vi "calculator.vi"() -> ()   [LabVIEW 2019]
panel:
  in  "Decimal Point Places":i16
  out "Previous Display":string
  in  ".":bool
  in  "=":bool
  in  "Clear":bool
  in  "Exit":bool
  out "Current Display":string
  in  "+":bool
  in  "-":bool
  in  "/":bool
  in  "x":bool
  in  "9":bool
  in  "8":bool
  in  "7":bool
  in  "6":bool
  in  "5":bool
  in  "4":bool
  in  "3":bool
  in  "0":bool
  in  "2":bool
  in  "1":bool
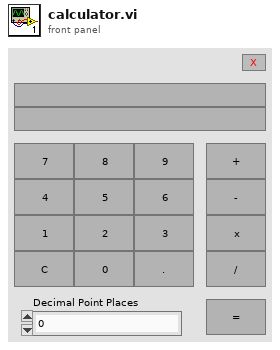
[diagram p1: front panel]
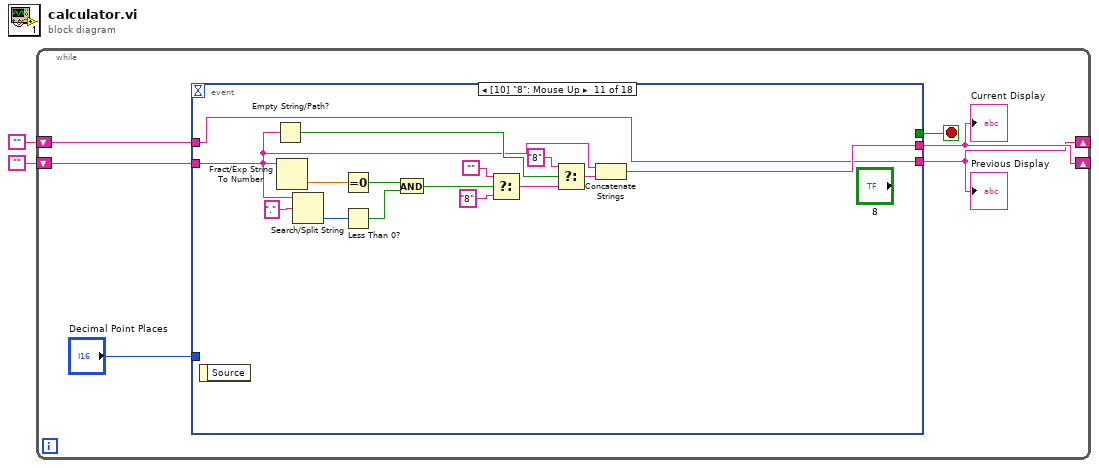
[diagram p0: block diagram]
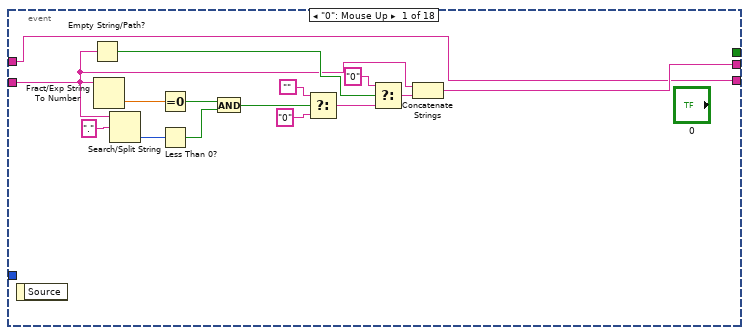
[diagram p2: hidden frame]
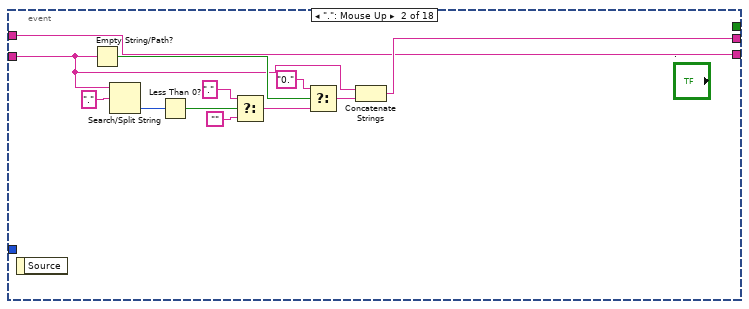
[diagram p3: hidden frame]
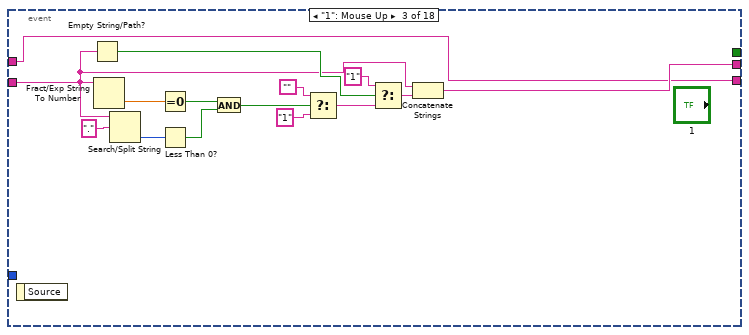
[diagram p4: hidden frame]
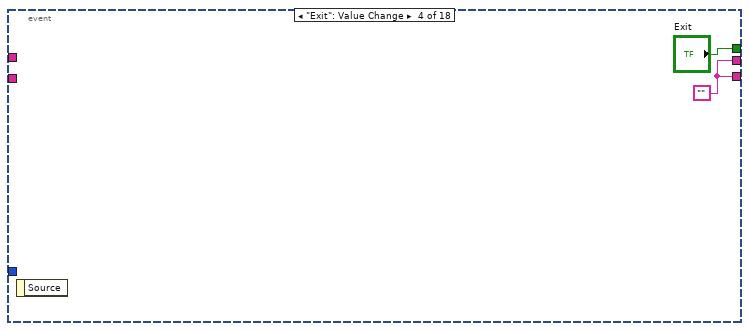
[diagram p5: hidden frame]
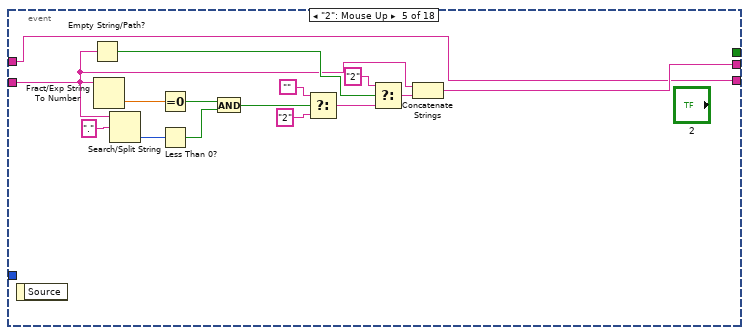
[diagram p6: hidden frame]
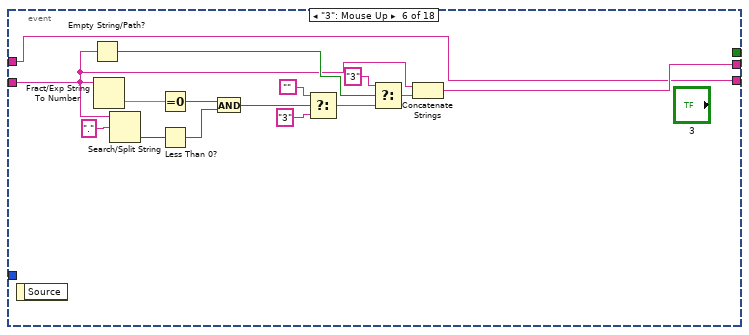
[diagram p7: hidden frame]
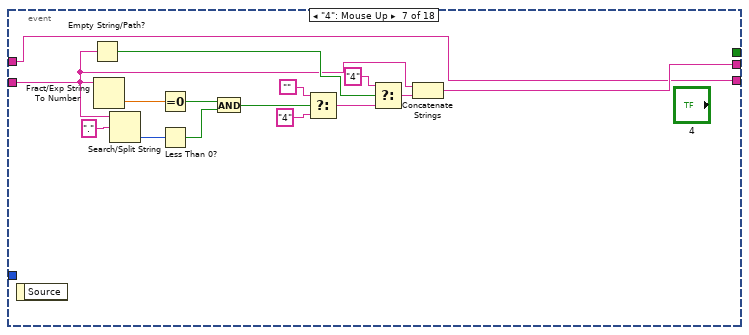
[diagram p8: hidden frame]
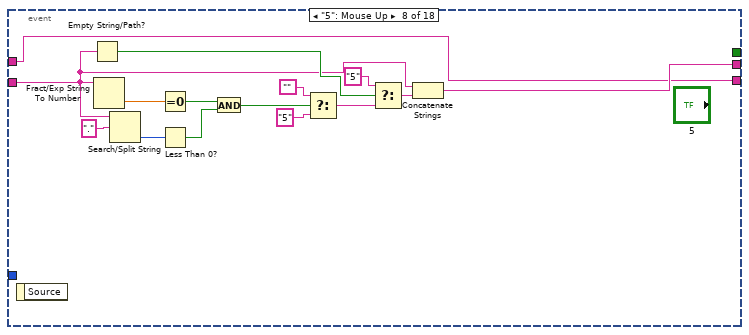
[diagram p9: hidden frame]
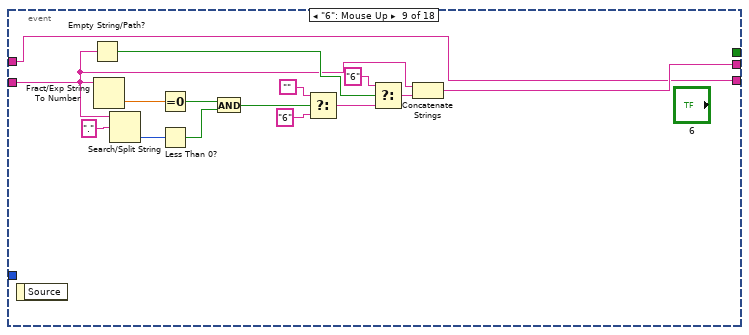
[diagram p10: hidden frame]
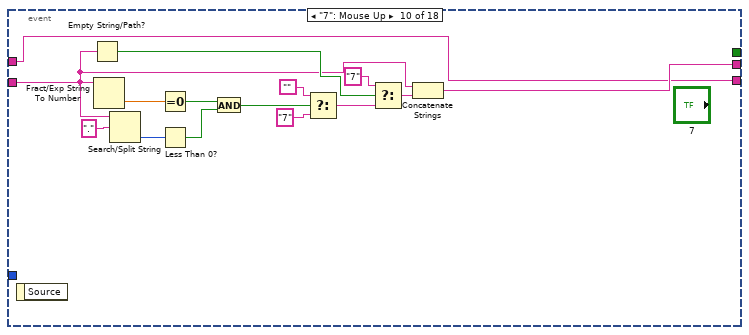
[diagram p11: hidden frame]
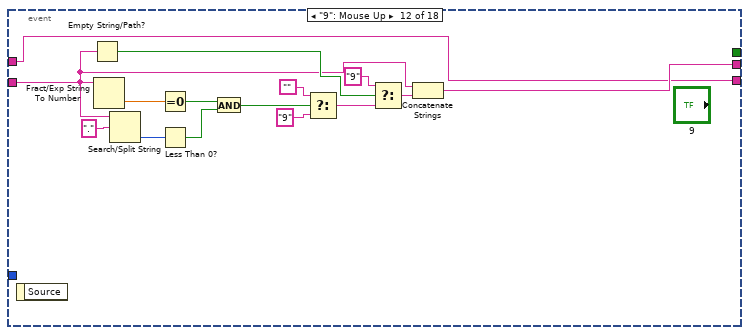
[diagram p12: hidden frame]
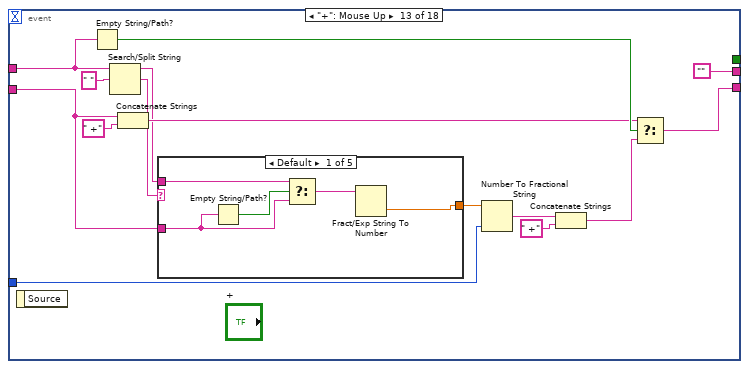
[diagram p13: hidden frame]
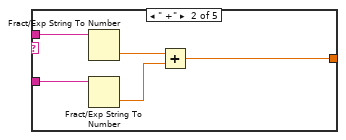
[diagram p14: hidden frame]
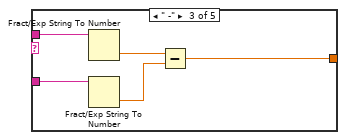
[diagram p15: hidden frame]
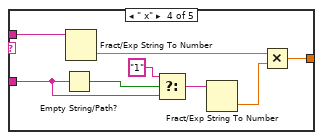
[diagram p16: hidden frame]
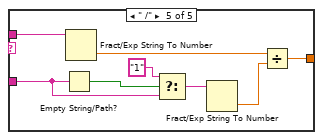
[diagram p17: hidden frame]
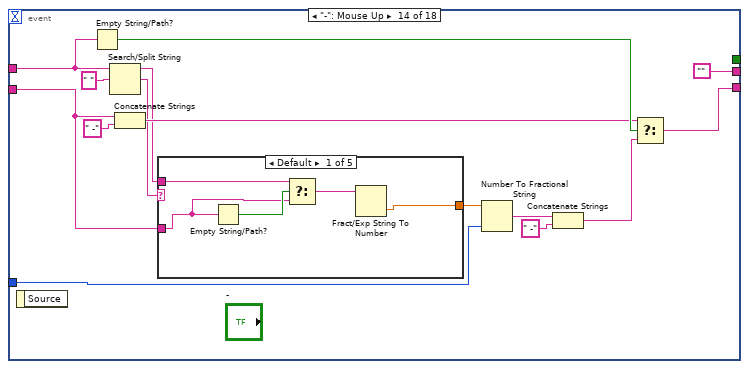
[diagram p18: hidden frame]
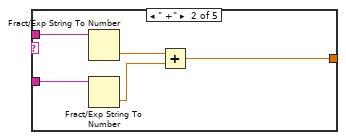
[diagram p19: hidden frame]
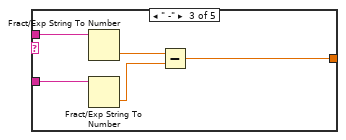
[diagram p20: hidden frame]
diagram:
  n1 = while {
    shift-right: [w8] -> _
    shift-left: "" -> [w7]
    shift-right: [w5] -> _
    shift-left: "" -> [w4]
    stop <- w6 stop-if-true
    n2 = event shown="[10] \"8\": Mouse Up" {
      selector: _ -> [_ _ _ _ _ _ _ _ _ _ _ _ _ _ _ _ _ _]
      dyn-events: _ -> [_ _ _ _ _ _ _ _ _ _ _ _ _ _ _ _ _ _]
      timeout: _ -> [_ _ _ _ _ _ _ _ _ _ _ _ _ _ _ _ _ _]
      tunnel: [w17 w27 w44 w51 w60 w75 w90 w105 w120 w135 w150 w165 "" "" "" "" "" w401] -> w8
      tunnel: w7 -> [w14 w28 w38 _ w55 w70 w85 w100 w115 w130 w145 w160 w174 w223 w271 w313 w358 _]
      tunnel: [_ _ _ "Exit" _ _ _ _ _ _ _ _ _ _ _ _ _ _] -> w6
      tunnel: [w15 w24 w42 w51 w59 w74 w89 w104 w119 w134 w149 w164 w184 w228 w270 w320 w360 w401] -> w5
      tunnel: w4 -> [w15 w24 w42 _ w59 w74 w89 w104 w119 w134 w149 w164 w183 w229 w272 w321 w359 _]
      tunnel: "Decimal Point Places" -> [_ _ _ _ _ _ _ _ _ _ _ _ w173 w219 w265 w311 w357 _]
      event "0": Mouse Up {
        n3 = event-data() -> ()  [unwired: 1 in, 1 out]
        n4 = Empty String/Path?(string/path=w14) -> (empty?=w23:bool)
        n5 = Fract/Exp String To Number(string=w14) -> (number=w21:dbl)  [unwired: 3 in, 1 out]
        n6 = Search/Split String(string=w14, search string/char (-)=".") -> (offset of match=w12:i32)  [unwired: 1 in, 2 out]
        n7 = Equal To 0?(x=w21) -> (x = 0?=w11:bool)
        n8 = Less Than 0?(x=w12) -> (x < 0?=w10:bool)
        n9 = And(x=w11, y=w10) -> (x .and. y?=w9:bool)
        n10 = Select(t="", s=w9, f="0") -> (s? t:f=w18:string)
        n11 = Select(t="0", s=w23, f=w18) -> (s? t:f=w16:string)
        n12 = Concatenate Strings(w14, w16) -> (w17:string)
      }
      event ".": Mouse Up {
        n13 = event-data() -> ()  [unwired: 1 in, 1 out]
        n14 = Empty String/Path?(string/path=w28) -> (empty?=w35:bool)
        n15 = Search/Split String(string=w28, search string/char (-)=".") -> (offset of match=w32:i32)  [unwired: 1 in, 2 out]
        n16 = Less Than 0?(x=w32) -> (x < 0?=w31:bool)
        n17 = Select(t=".", s=w31, f="") -> (s? t:f=w30:string)
        n18 = Select(t="0.", s=w35, f=w30) -> (s? t:f=w29:string)
        n19 = Concatenate Strings(w28, w29) -> (w27:string)
      }
      event "1": Mouse Up {
        n20 = event-data() -> ()  [unwired: 1 in, 1 out]
        n21 = Empty String/Path?(string/path=w38) -> (empty?=w50:bool)
        n22 = Fract/Exp String To Number(string=w38) -> (number=w49:dbl)  [unwired: 3 in, 1 out]
        n23 = Search/Split String(string=w38, search string/char (-)=".") -> (offset of match=w40:i32)  [unwired: 1 in, 2 out]
        n24 = Equal To 0?(x=w49) -> (x = 0?=w37:bool)
        n25 = Less Than 0?(x=w40) -> (x < 0?=w39:bool)
        n26 = And(x=w37, y=w39) -> (x .and. y?=w36:bool)
        n27 = Select(t="", s=w36, f="1") -> (s? t:f=w46:string)
        n28 = Select(t="1", s=w50, f=w46) -> (s? t:f=w43:string)
        n29 = Concatenate Strings(w38, w43) -> (w44:string)
      }
      event "Exit": Value Change {
        w51 = ""
        n30 = event-data() -> ()  [unwired: 1 in, 1 out]
      }
      event "2": Mouse Up {
        n31 = event-data() -> ()  [unwired: 1 in, 1 out]
        n32 = Empty String/Path?(string/path=w55) -> (empty?=w67:bool)
        n33 = Fract/Exp String To Number(string=w55) -> (number=w65:dbl)  [unwired: 3 in, 1 out]
        n34 = Search/Split String(string=w55, search string/char (-)=".") -> (offset of match=w57:i32)  [unwired: 1 in, 2 out]
        n35 = Equal To 0?(x=w65) -> (x = 0?=w54:bool)
        n36 = Less Than 0?(x=w57) -> (x < 0?=w56:bool)
        n37 = And(x=w54, y=w56) -> (x .and. y?=w53:bool)
        n38 = Select(t="", s=w53, f="2") -> (s? t:f=w62:string)
        n39 = Select(t="2", s=w67, f=w62) -> (s? t:f=w61:string)
        n40 = Concatenate Strings(w55, w61) -> (w60:string)
      }
      event "3": Mouse Up {
        n41 = event-data() -> ()  [unwired: 1 in, 1 out]
        n42 = Empty String/Path?(string/path=w70) -> (empty?=w82:bool)
        n43 = Fract/Exp String To Number(string=w70) -> (number=w80:dbl)  [unwired: 3 in, 1 out]
        n44 = Search/Split String(string=w70, search string/char (-)=".") -> (offset of match=w72:i32)  [unwired: 1 in, 2 out]
        n45 = Equal To 0?(x=w80) -> (x = 0?=w69:bool)
        n46 = Less Than 0?(x=w72) -> (x < 0?=w71:bool)
        n47 = And(x=w69, y=w71) -> (x .and. y?=w68:bool)
        n48 = Select(t="", s=w68, f="3") -> (s? t:f=w77:string)
        n49 = Select(t="3", s=w82, f=w77) -> (s? t:f=w76:string)
        n50 = Concatenate Strings(w70, w76) -> (w75:string)
      }
      event "4": Mouse Up {
        n51 = event-data() -> ()  [unwired: 1 in, 1 out]
        n52 = Empty String/Path?(string/path=w85) -> (empty?=w97:bool)
        n53 = Fract/Exp String To Number(string=w85) -> (number=w95:dbl)  [unwired: 3 in, 1 out]
        n54 = Search/Split String(string=w85, search string/char (-)=".") -> (offset of match=w87:i32)  [unwired: 1 in, 2 out]
        n55 = Equal To 0?(x=w95) -> (x = 0?=w84:bool)
        n56 = Less Than 0?(x=w87) -> (x < 0?=w86:bool)
        n57 = And(x=w84, y=w86) -> (x .and. y?=w83:bool)
        n58 = Select(t="", s=w83, f="4") -> (s? t:f=w92:string)
        n59 = Select(t="4", s=w97, f=w92) -> (s? t:f=w91:string)
        n60 = Concatenate Strings(w85, w91) -> (w90:string)
      }
      event "5": Mouse Up {
        n61 = event-data() -> ()  [unwired: 1 in, 1 out]
        n62 = Empty String/Path?(string/path=w100) -> (empty?=w112:bool)
        n63 = Fract/Exp String To Number(string=w100) -> (number=w110:dbl)  [unwired: 3 in, 1 out]
        n64 = Search/Split String(string=w100, search string/char (-)=".") -> (offset of match=w102:i32)  [unwired: 1 in, 2 out]
        n65 = Equal To 0?(x=w110) -> (x = 0?=w99:bool)
        n66 = Less Than 0?(x=w102) -> (x < 0?=w101:bool)
        n67 = And(x=w99, y=w101) -> (x .and. y?=w98:bool)
        n68 = Select(t="", s=w98, f="5") -> (s? t:f=w107:string)
        n69 = Select(t="5", s=w112, f=w107) -> (s? t:f=w106:string)
        n70 = Concatenate Strings(w100, w106) -> (w105:string)
      }
      event "6": Mouse Up {
        n71 = event-data() -> ()  [unwired: 1 in, 1 out]
        n72 = Empty String/Path?(string/path=w115) -> (empty?=w127:bool)
        n73 = Fract/Exp String To Number(string=w115) -> (number=w125:dbl)  [unwired: 3 in, 1 out]
        n74 = Search/Split String(string=w115, search string/char (-)=".") -> (offset of match=w117:i32)  [unwired: 1 in, 2 out]
        n75 = Equal To 0?(x=w125) -> (x = 0?=w114:bool)
        n76 = Less Than 0?(x=w117) -> (x < 0?=w116:bool)
        n77 = And(x=w114, y=w116) -> (x .and. y?=w113:bool)
        n78 = Select(t="", s=w113, f="6") -> (s? t:f=w122:string)
        n79 = Select(t="6", s=w127, f=w122) -> (s? t:f=w121:string)
        n80 = Concatenate Strings(w115, w121) -> (w120:string)
      }
      event "7": Mouse Up {
        n81 = event-data() -> ()  [unwired: 1 in, 1 out]
        n82 = Empty String/Path?(string/path=w130) -> (empty?=w142:bool)
        n83 = Fract/Exp String To Number(string=w130) -> (number=w140:dbl)  [unwired: 3 in, 1 out]
        n84 = Search/Split String(string=w130, search string/char (-)=".") -> (offset of match=w132:i32)  [unwired: 1 in, 2 out]
        n85 = Equal To 0?(x=w140) -> (x = 0?=w129:bool)
        n86 = Less Than 0?(x=w132) -> (x < 0?=w131:bool)
        n87 = And(x=w129, y=w131) -> (x .and. y?=w128:bool)
        n88 = Select(t="", s=w128, f="7") -> (s? t:f=w137:string)
        n89 = Select(t="7", s=w142, f=w137) -> (s? t:f=w136:string)
        n90 = Concatenate Strings(w130, w136) -> (w135:string)
      }
      event "8": Mouse Up {
        n91 = event-data() -> ()  [unwired: 1 in, 1 out]
        n92 = Empty String/Path?(string/path=w145) -> (empty?=w157:bool)
        n93 = Fract/Exp String To Number(string=w145) -> (number=w155:dbl)  [unwired: 3 in, 1 out]
        n94 = Search/Split String(string=w145, search string/char (-)=".") -> (offset of match=w147:i32)  [unwired: 1 in, 2 out]
        n95 = Equal To 0?(x=w155) -> (x = 0?=w144:bool)
        n96 = Less Than 0?(x=w147) -> (x < 0?=w146:bool)
        n97 = And(x=w144, y=w146) -> (x .and. y?=w143:bool)
        n98 = Select(t="", s=w143, f="8") -> (s? t:f=w152:string)
        n99 = Select(t="8", s=w157, f=w152) -> (s? t:f=w151:string)
        n100 = Concatenate Strings(w145, w151) -> (w150:string)
      }
      event "9": Mouse Up {
        n101 = event-data() -> ()  [unwired: 1 in, 1 out]
        n102 = Empty String/Path?(string/path=w160) -> (empty?=w172:bool)
        n103 = Fract/Exp String To Number(string=w160) -> (number=w170:dbl)  [unwired: 3 in, 1 out]
        n104 = Search/Split String(string=w160, search string/char (-)=".") -> (offset of match=w162:i32)  [unwired: 1 in, 2 out]
        n105 = Equal To 0?(x=w170) -> (x = 0?=w159:bool)
        n106 = Less Than 0?(x=w162) -> (x < 0?=w161:bool)
        n107 = And(x=w159, y=w161) -> (x .and. y?=w158:bool)
        n108 = Select(t="", s=w158, f="9") -> (s? t:f=w167:string)
        n109 = Select(t="9", s=w172, f=w167) -> (s? t:f=w166:string)
        n110 = Concatenate Strings(w160, w166) -> (w165:string)
      }
      event "+": Mouse Up {
        n111 = event-data() -> ()  [unwired: 1 in, 1 out]
        n112 = Empty String/Path?(string/path=w183) -> (empty?=w187:bool)
        n113 = Search/Split String(string=w183, search string/char (-)=" ") -> (substring before match=w176:string, match + rest of string=w175:string)  [unwired: 1 in, 1 out]
        n114 = Concatenate Strings(w174, " +" ("string")) -> (w185:string)
        n115 = case shown="Default" w175 {
          tunnel: w176 -> [w190 w197 w200 w208 w216]
          tunnel: w174 -> [w188 w196 w199 w204 w214]
          tunnel: [w192 w193 w198 w207 w215] -> w177
          frame Default {
            n116 = Empty String/Path?(string/path=w188) -> (empty?=w191:bool)
            n117 = Select(t=w190, s=w191, f=w188) -> (s? t:f=w189:string)
            n118 = Fract/Exp String To Number(string=w189) -> (number=w192:dbl)  [unwired: 3 in, 1 out]
          }
          frame " +" {
            n119 = Fract/Exp String To Number(string=w197) -> (number=w195:dbl)  [unwired: 3 in, 1 out]
            n120 = Fract/Exp String To Number(string=w196) -> (number=w194:dbl)  [unwired: 3 in, 1 out]
            n121 = Add(x=w195, y=w194) -> (x+y=w193:dbl)
          }
          frame " -" {
            n122 = Fract/Exp String To Number(string=w200) -> (number=w202:dbl)  [unwired: 3 in, 1 out]
            n123 = Fract/Exp String To Number(string=w199) -> (number=w201:dbl)  [unwired: 3 in, 1 out]
            n124 = Subtract(x=w202, y=w201) -> (x-y=w198:dbl)
          }
          frame " x" {
            n125 = Empty String/Path?(string/path=w204) -> (empty?=w206:bool)
            n126 = Fract/Exp String To Number(string=w208) -> (number=w210:dbl)  [unwired: 3 in, 1 out]
            n127 = Select(t="1", s=w206, f=w204) -> (s? t:f=w203:string)
            n128 = Fract/Exp String To Number(string=w203) -> (number=w209:dbl)  [unwired: 3 in, 1 out]
            n129 = Multiply(x=w210, y=w209) -> (x*y=w207:dbl)
          }
          frame " /" {
            n130 = Empty String/Path?(string/path=w214) -> (empty?=w213:bool)
            n131 = Fract/Exp String To Number(string=w216) -> (number=w218:dbl)  [unwired: 3 in, 1 out]
            n132 = Select(t="1", s=w213, f=w214) -> (s? t:f=w211:string)
            n133 = Fract/Exp String To Number(string=w211) -> (number=w217:dbl)  [unwired: 3 in, 1 out]
            n134 = Divide(x=w218, y=w217) -> (x/y=w215:dbl)
          }
        }
        n135 = Number To Fractional String(number=w177, precision (6)=w173) -> (F-format string=w179:string)  [unwired: 2 in]
        n136 = Concatenate Strings(w179, " +" ("string")) -> (w178:string)
        n137 = Select(t=w185, s=w187, f=w178) -> (s? t:f=w184:string)
      }
      event "-": Mouse Up {
        n138 = event-data() -> ()  [unwired: 1 in, 1 out]
        n139 = Empty String/Path?(string/path=w229) -> (empty?=w233:bool)
        n140 = Search/Split String(string=w229, search string/char (-)=" ") -> (substring before match=w221:string, match + rest of string=w222:string)  [unwired: 1 in, 1 out]
        n141 = Concatenate Strings(w223, " -" ("string")) -> (w231:string)
        n142 = case shown="Default" w222 {
          tunnel: w221 -> [w235 w243 w246 w254 w262]
          tunnel: w223 -> [w236 w242 w245 w250 w260]
          tunnel: [w238 w239 w244 w253 w261] -> w220
          frame Default {
            n143 = Empty String/Path?(string/path=w236) -> (empty?=w237:bool)
            n144 = Select(t=w235, s=w237, f=w236) -> (s? t:f=w234:string)
            n145 = Fract/Exp String To Number(string=w234) -> (number=w238:dbl)  [unwired: 3 in, 1 out]
          }
          frame " +" {
            n146 = Fract/Exp String To Number(string=w243) -> (number=w241:dbl)  [unwired: 3 in, 1 out]
            n147 = Fract/Exp String To Number(string=w242) -> (number=w240:dbl)  [unwired: 3 in, 1 out]
            n148 = Add(x=w241, y=w240) -> (x+y=w239:dbl)
          }
          frame " -" {
            n149 = Fract/Exp String To Number(string=w246) -> (number=w248:dbl)  [unwired: 3 in, 1 out]
            n150 = Fract/Exp String To Number(string=w245) -> (number=w247:dbl)  [unwired: 3 in, 1 out]
            n151 = Subtract(x=w248, y=w247) -> (x-y=w244:dbl)
          }
          frame " x" {
            n152 = Empty String/Path?(string/path=w250) -> (empty?=w252:bool)
            n153 = Fract/Exp String To Number(string=w254) -> (number=w256:dbl)  [unwired: 3 in, 1 out]
            n154 = Select(t="1", s=w252, f=w250) -> (s? t:f=w249:string)
            n155 = Fract/Exp String To Number(string=w249) -> (number=w255:dbl)  [unwired: 3 in, 1 out]
            n156 = Multiply(x=w256, y=w255) -> (x*y=w253:dbl)
          }
          frame " /" {
            n157 = Empty String/Path?(string/path=w260) -> (empty?=w259:bool)
            n158 = Fract/Exp String To Number(string=w262) -> (number=w264:dbl)  [unwired: 3 in, 1 out]
            n159 = Select(t="1", s=w259, f=w260) -> (s? t:f=w257:string)
            n160 = Fract/Exp String To Number(string=w257) -> (number=w263:dbl)  [unwired: 3 in, 1 out]
            n161 = Divide(x=w264, y=w263) -> (x/y=w261:dbl)
          }
        }
        n162 = Number To Fractional String(number=w220, precision (6)=w219) -> (F-format string=w226:string)  [unwired: 2 in]
        n163 = Concatenate Strings(w226, " -" ("string")) -> (w224:string)
        n164 = Select(t=w231, s=w233, f=w224) -> (s? t:f=w228:string)
      }
      event "x": Mouse Up {
        n165 = event-data() -> ()  [unwired: 1 in, 1 out]
        n166 = Empty String/Path?(string/path=w272) -> (empty?=w279:bool)
        n167 = Search/Split String(string=w272, search string/char (-)=" ") -> (substring before match=w274:string, match + rest of string=w275:string)  [unwired: 1 in, 1 out]
        n168 = Concatenate Strings(w271, " x" ("string")) -> (w277:string)
        n169 = case shown="Default" w275 {
          tunnel: w274 -> [w281 w289 w292 w300 w308]
          tunnel: w271 -> [w282 w288 w291 w296 w306]
          tunnel: [w284 w285 w290 w299 w307] -> w273
          frame Default {
            n170 = Empty String/Path?(string/path=w282) -> (empty?=w283:bool)
            n171 = Select(t=w281, s=w283, f=w282) -> (s? t:f=w280:string)
            n172 = Fract/Exp String To Number(string=w280) -> (number=w284:dbl)  [unwired: 3 in, 1 out]
          }
          frame " +" {
            n173 = Fract/Exp String To Number(string=w289) -> (number=w287:dbl)  [unwired: 3 in, 1 out]
            n174 = Fract/Exp String To Number(string=w288) -> (number=w286:dbl)  [unwired: 3 in, 1 out]
            n175 = Add(x=w287, y=w286) -> (x+y=w285:dbl)
          }
          frame " -" {
            n176 = Fract/Exp String To Number(string=w292) -> (number=w294:dbl)  [unwired: 3 in, 1 out]
            n177 = Fract/Exp String To Number(string=w291) -> (number=w293:dbl)  [unwired: 3 in, 1 out]
            n178 = Subtract(x=w294, y=w293) -> (x-y=w290:dbl)
          }
          frame " x" {
            n179 = Empty String/Path?(string/path=w296) -> (empty?=w298:bool)
            n180 = Fract/Exp String To Number(string=w300) -> (number=w302:dbl)  [unwired: 3 in, 1 out]
            n181 = Select(t="1", s=w298, f=w296) -> (s? t:f=w295:string)
            n182 = Fract/Exp String To Number(string=w295) -> (number=w301:dbl)  [unwired: 3 in, 1 out]
            n183 = Multiply(x=w302, y=w301) -> (x*y=w299:dbl)
          }
          frame " /" {
            n184 = Empty String/Path?(string/path=w306) -> (empty?=w305:bool)
            n185 = Fract/Exp String To Number(string=w308) -> (number=w310:dbl)  [unwired: 3 in, 1 out]
            n186 = Select(t="1", s=w305, f=w306) -> (s? t:f=w303:string)
            n187 = Fract/Exp String To Number(string=w303) -> (number=w309:dbl)  [unwired: 3 in, 1 out]
            n188 = Divide(x=w310, y=w309) -> (x/y=w307:dbl)
          }
        }
        n189 = Number To Fractional String(number=w273, precision (6)=w265) -> (F-format string=w268:string)  [unwired: 2 in]
        n190 = Concatenate Strings(w268, " x" ("string")) -> (w266:string)
        n191 = Select(t=w277, s=w279, f=w266) -> (s? t:f=w270:string)
      }
      event "/": Mouse Up {
        n192 = event-data() -> ()  [unwired: 1 in, 1 out]
        n193 = Empty String/Path?(string/path=w321) -> (empty?=w325:bool)
        n194 = Search/Split String(string=w321, search string/char (-)=" ") -> (substring before match=w315:string, match + rest of string=w314:string)  [unwired: 1 in, 1 out]
        n195 = Concatenate Strings(w313, " /" ("string")) -> (w323:string)
        n196 = case shown="Default" w314 {
          tunnel: w315 -> [w327 w335 w338 w346 w354]
          tunnel: w313 -> [w328 w334 w337 w342 w352]
          tunnel: [w330 w331 w336 w345 w353] -> w312
          frame Default {
            n197 = Empty String/Path?(string/path=w328) -> (empty?=w329:bool)
            n198 = Select(t=w327, s=w329, f=w328) -> (s? t:f=w326:string)
            n199 = Fract/Exp String To Number(string=w326) -> (number=w330:dbl)  [unwired: 3 in, 1 out]
          }
          frame " +" {
            n200 = Fract/Exp String To Number(string=w335) -> (number=w333:dbl)  [unwired: 3 in, 1 out]
            n201 = Fract/Exp String To Number(string=w334) -> (number=w332:dbl)  [unwired: 3 in, 1 out]
            n202 = Add(x=w333, y=w332) -> (x+y=w331:dbl)
          }
          frame " -" {
            n203 = Fract/Exp String To Number(string=w338) -> (number=w340:dbl)  [unwired: 3 in, 1 out]
            n204 = Fract/Exp String To Number(string=w337) -> (number=w339:dbl)  [unwired: 3 in, 1 out]
            n205 = Subtract(x=w340, y=w339) -> (x-y=w336:dbl)
          }
          frame " x" {
            n206 = Empty String/Path?(string/path=w342) -> (empty?=w344:bool)
            n207 = Fract/Exp String To Number(string=w346) -> (number=w348:dbl)  [unwired: 3 in, 1 out]
            n208 = Select(t="1", s=w344, f=w342) -> (s? t:f=w341:string)
            n209 = Fract/Exp String To Number(string=w341) -> (number=w347:dbl)  [unwired: 3 in, 1 out]
            n210 = Multiply(x=w348, y=w347) -> (x*y=w345:dbl)
          }
          frame " /" {
            n211 = Empty String/Path?(string/path=w352) -> (empty?=w351:bool)
            n212 = Fract/Exp String To Number(string=w354) -> (number=w356:dbl)  [unwired: 3 in, 1 out]
            n213 = Select(t="1", s=w351, f=w352) -> (s? t:f=w349:string)
            n214 = Fract/Exp String To Number(string=w349) -> (number=w355:dbl)  [unwired: 3 in, 1 out]
            n215 = Divide(x=w356, y=w355) -> (x/y=w353:dbl)
          }
        }
        n216 = Number To Fractional String(number=w312, precision (6)=w311) -> (F-format string=w318:string)  [unwired: 2 in]
        n217 = Concatenate Strings(w318, " /" ("string")) -> (w316:string)
        n218 = Select(t=w323, s=w325, f=w316) -> (s? t:f=w320:string)
      }
      event "=": Mouse Up {
        n219 = event-data() -> ()  [unwired: 1 in, 1 out]
        n220 = Empty String/Path?(string/path=w359) -> (empty?=w369:bool)
        n221 = Search/Split String(string=w359, search string/char (-)=" ") -> (substring before match=w363:string, match + rest of string=w362:string)  [unwired: 1 in, 1 out]
        n222 = case shown="Default" w362 {
          tunnel: w363 -> [w372 w379 w382 w390 w398]
          tunnel: w358 -> [w371 w378 w381 w386 w396]
          tunnel: [w374 w375 w380 w389 w397] -> w364
          frame Default {
            n223 = Empty String/Path?(string/path=w371) -> (empty?=w373:bool)
            n224 = Select(t=w372, s=w373, f=w371) -> (s? t:f=w370:string)
            n225 = Fract/Exp String To Number(string=w370) -> (number=w374:dbl)  [unwired: 3 in, 1 out]
          }
          frame " +" {
            n226 = Fract/Exp String To Number(string=w379) -> (number=w377:dbl)  [unwired: 3 in, 1 out]
            n227 = Fract/Exp String To Number(string=w378) -> (number=w376:dbl)  [unwired: 3 in, 1 out]
            n228 = Add(x=w377, y=w376) -> (x+y=w375:dbl)
          }
          frame " -" {
            n229 = Fract/Exp String To Number(string=w382) -> (number=w384:dbl)  [unwired: 3 in, 1 out]
            n230 = Fract/Exp String To Number(string=w381) -> (number=w383:dbl)  [unwired: 3 in, 1 out]
            n231 = Subtract(x=w384, y=w383) -> (x-y=w380:dbl)
          }
          frame " x" {
            n232 = Empty String/Path?(string/path=w386) -> (empty?=w388:bool)
            n233 = Fract/Exp String To Number(string=w390) -> (number=w392:dbl)  [unwired: 3 in, 1 out]
            n234 = Select(t="1", s=w388, f=w386) -> (s? t:f=w385:string)
            n235 = Fract/Exp String To Number(string=w385) -> (number=w391:dbl)  [unwired: 3 in, 1 out]
            n236 = Multiply(x=w392, y=w391) -> (x*y=w389:dbl)
          }
          frame " /" {
            n237 = Empty String/Path?(string/path=w396) -> (empty?=w395:bool)
            n238 = Fract/Exp String To Number(string=w398) -> (number=w400:dbl)  [unwired: 3 in, 1 out]
            n239 = Select(t="1", s=w395, f=w396) -> (s? t:f=w393:string)
            n240 = Fract/Exp String To Number(string=w393) -> (number=w399:dbl)  [unwired: 3 in, 1 out]
            n241 = Divide(x=w400, y=w399) -> (x/y=w397:dbl)
          }
        }
        n242 = Number To Fractional String(number=w364, precision (6)=w357) -> (F-format string=w366:string)  [unwired: 2 in]
        n243 = Concatenate Strings(w366, "" ("string")) -> (w365:string)
        n244 = Select(t=w358, s=w369, f=w365) -> (s? t:f=w360:string)
      }
      event "Clear": Mouse Up {
        w401 = ""
        n245 = event-data() -> ()  [unwired: 1 in, 1 out]
      }
    }
    "Current Display" <- w8
    "Previous Display" <- w5
  }
